vi "cw_1_7.vi"() -> ()   [LabVIEW 2022 SP3]
panel:
  out "Decimal":dbl
  out "f(A,B,C)":bool[](array[boolean])
  out "Possible States":string[][](array[string])
  in  "Array":bool[](array[boolean])=[FALSE, FALSE, FALSE, TRUE, TRUE, TRUE, FALSE, FALSE, FALSE]
  out "f(A,B,C)":bool
  out "Boolean 5":bool
  out "Boolean 4":bool
  out "Boolean 4":bool
  in  "C":bool
  in  "B":bool
  in  "A":bool
  out "Result True?":bool
  in  "C":bool
  in  "B":bool
  in  "A":bool
  # "Version A (programmable truth table)"
  # "Version B (fixed truth table)"
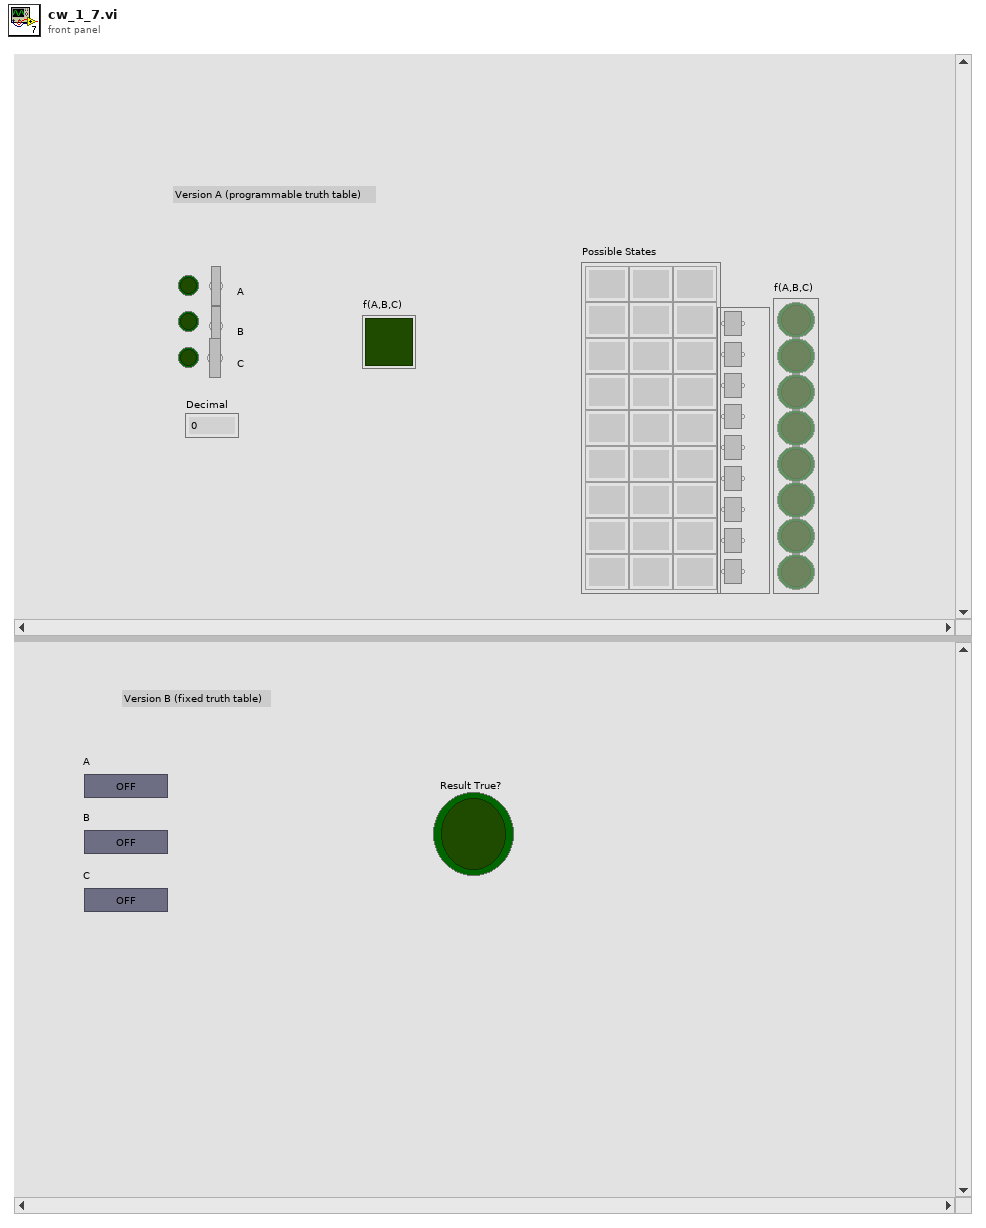
[diagram p1: front panel]
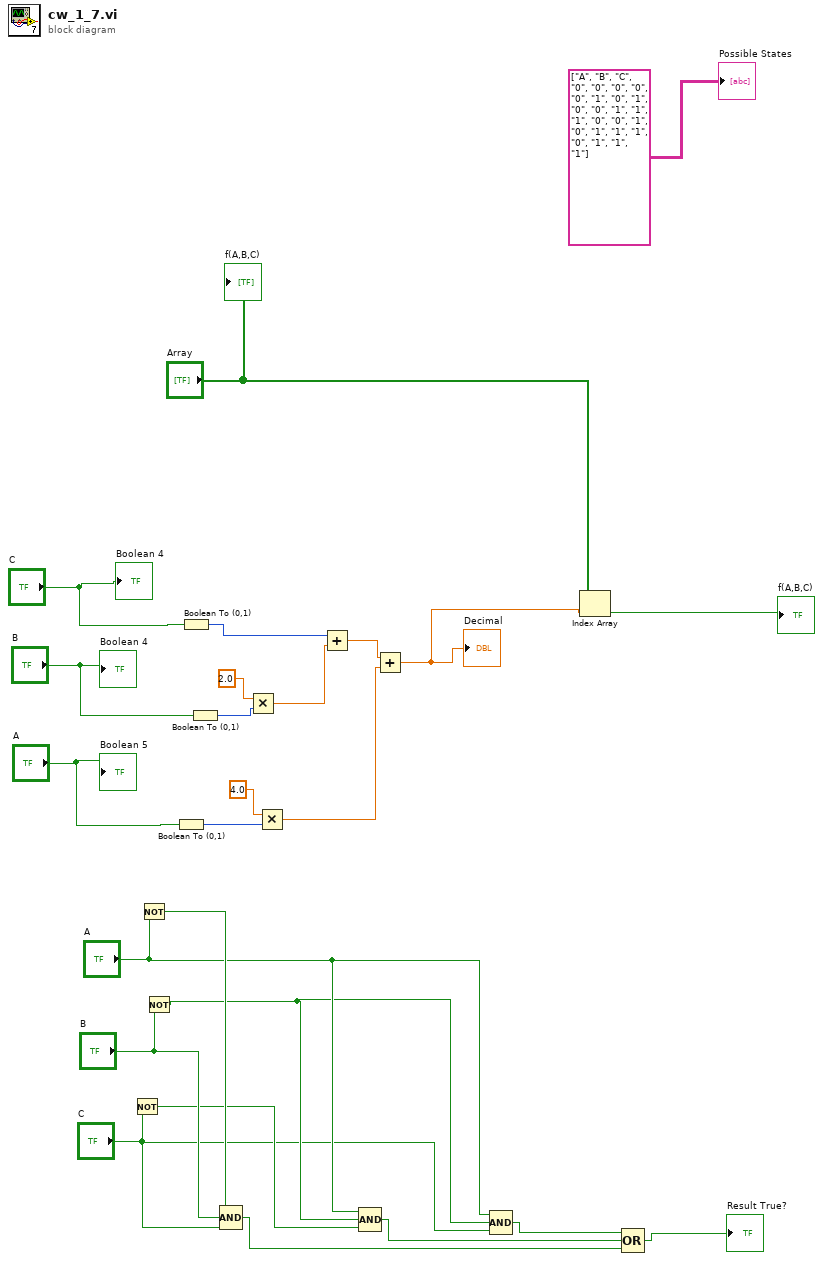
[diagram p0: block diagram]
diagram:
  n1 = Not(x="C") -> (.not. x?=w11:bool)
  n2 = Not(x="A") -> (.not. x?=w13:bool)
  n3 = Not(x="B") -> (.not. x?=w9:bool)
  n4 = Boolean To (0,1)(Boolean="A") -> (0, 1=w21:i16)
  n5 = Boolean To (0,1)(Boolean="C") -> (0, 1=w25:i16)
  n6 = Boolean To (0,1)(Boolean="B") -> (0, 1=w20:i16)
  n7 = Compound Arithmetic op=AND(w13, "B", "C") -> (w5:bool)
  n8 = Multiply(x=2.0, y=w20) -> (x*y=w19:dbl)
  n9 = Multiply(x=4.0 ("y"), y=w21) -> (x*y=w18:dbl)
  n10 = Add(x=w25, y=w19) -> (x+y=w17:dbl)
  n11 = Compound Arithmetic op=AND("A", w9, w11) -> (w6:bool)
  n12 = Add(x=w17, y=w18) -> (x+y=w15:dbl)
  "Decimal" <- w15
  n13 = Compound Arithmetic op=AND("A", w9, "C") -> (w7:bool)
  n14 = Index Array(array="Array", index=w15) -> (element=→"f(A,B,C)":bool)
  n15 = Compound Arithmetic op=OR(w7, w6, w5) -> (→"Result True?":bool)
  "Boolean 4" <- "C"
  "Boolean 4" <- "B"
  "Boolean 5" <- "A"
  "f(A,B,C)" <- "Array"
  "Possible States" <- string[][] [["A", "B", "C"], ["0", "0", "0"], ["0", "0", "1"], ["0", "1", "0"], ["0", "1", "1"], ["1", "0", "0"], ["1", "0", "1"], ["1", "1", "0"], ["1", "1", "1"]] ("Possible States 2")
